vi "AutoHelper_Timeout.vi"(6 "Pass_Through_Time":dbl=-1.0 format="%33.4f", 9 "Timeout Sec":dbl, 11 "New Step":bool) -> (1 "Remaining":dbl, 3 "Timeout":bool)   [LabVIEW 2019, in "Trajectory_Library.lvlib"]
doc: "Implements a simplified state machine similar to a mechanical / electrical drum sequencer. When the Drum Sequencer is \"Ready\" and the \"Initiate\" input becomes TRUE,, the drum sequences through its set of steps from 1 to N. After each Step is executed it is followed by a wait. During the wait the Step output indicates \"Do Nothing\". The number of Steps is determined by the number of elements in the \"Step Times\" input array. Once all the steps have been executed, the Drum Sequencer cycles bac to wait for another initiate. \n\nThere is a Cancel input that interrupts the sequence, executes the Cancel Step, performs the cancel wait, and then returns to wait for an Initiate action. \n\nIf any of the Step Times, or Cancel times are negative, or there more than 32 steps, or less than 1 step an error is signaled. The drum sequencer selects the error state and stays there.\n\nInputs:\n\nOutputs:"
uses:
  Trajectory_Library.lvlib
  Util_GetTime_U32.vi
  Util_GetTime_U64.vi
  <vilib>/Utility/semaphor.llb/Obtain Semaphore Reference.vi
  Timer_Reset.vi
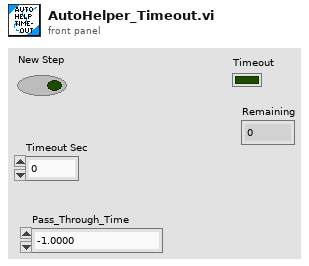
[diagram p1: front panel]
types:
  T1 = typedef "Trajectory_Library.lvlib/TIMER.ctl" = cluster{"StartTime":dbl, "Accumulated TIme":dbl, "Running":bool, "semaphore":T2}
  T2 = typedef "Semaphore RefNum" = refnum<k1>
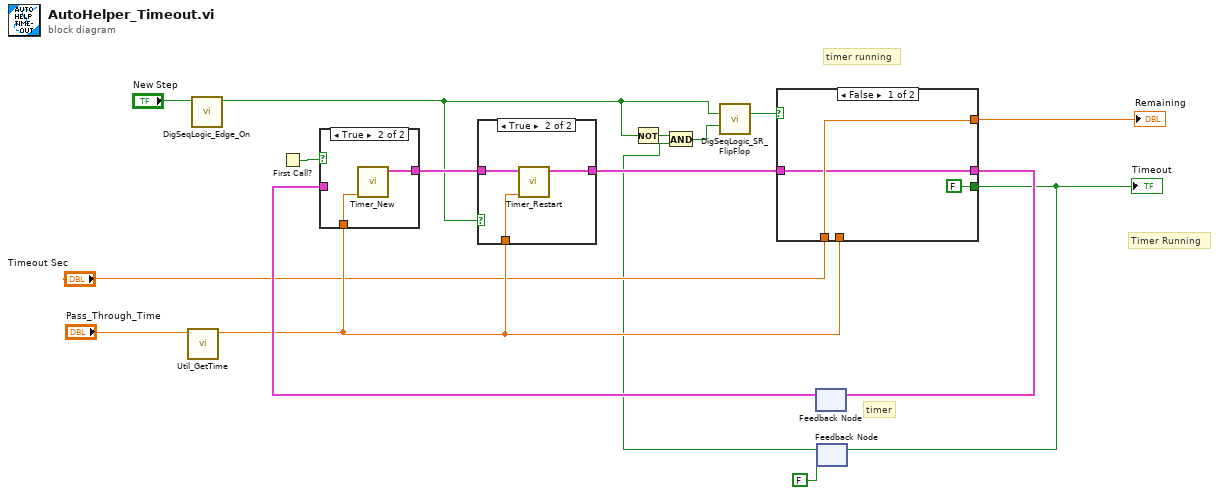
[diagram p0: block diagram]
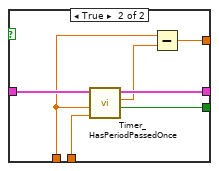
[diagram p2: hidden frame]
diagram:
  # "timer running"
  # "Timer Running"
  # "timer"
  n1 = call "Util_GetTime.vi"("Pass_Through_Time"="Pass_Through_Time") -> ("FPGA_Time_Seconds"=w11:dbl)  [unwired: 8 in, 2 out]
  n2 = call "DigSeqLogic_Edge_On.vi"("Input"="New Step") -> ("On Edge"=w5:bool)  [unwired: 10 in]
  n3 = First Call?() -> (First Call?: T/F=w15:bool)
  n4 = Not(x=w5) -> (.not. x?=w4:bool)
  n5 = feedback #1() -> (w14:T1)  [unwired: 1 in]
  n6 = case shown="True" w15 {
    tunnel: [w18 w20] -> w13
    tunnel: w11 -> [_ w19]
    tunnel: w14 -> [w18 _]
    frame False {
    }
    frame True {
      n7 = call "Timer_New.vi"("Pass_Through_Time"=w19) -> ("TIMER"=w20:T1)  [unwired: 10 in]
    }
  }
  n8 = case shown="True" w5 {
    tunnel: [w21 w24] -> w12
    tunnel: w13 -> [w21 w23]
    tunnel: w11 -> [_ w22]
    frame False {
    }
    frame True {
      n9 = call "Timer_Restart.vi"("Pass_Through_Time"=w22, "in Timer"=w23) -> ("out Timer"=w24:T1)  [unwired: 9 in]
    }
  }
  n10 = feedback #2(FALSE ("Expired")) -> (w2:bool)
  n11 = And(x=w4, y=w2) -> (x .and. y?=w3:bool)
  n12 = call "DigSeqLogic_SR_FlipFlop.vi"("Set"=w5, "Reset"=w3) -> ("Output"=w7:bool)  [unwired: 12 in, 1 out]
  n13 = case shown="False" w7 {
    tunnel: w12 -> [w26 w34]
    tunnel: w11 -> [_ w33]
    tunnel: [w26 w32] -> w10
    tunnel: "Timeout Sec" -> [w27 w31]
    tunnel: [w27 w29] -> w8
    tunnel: [FALSE ("Expired") w28] -> w6
    frame False {
    }
    frame True {
      n14 = call "Timer_HasPeriodPassedOnce.vi"("Pass_Through_Time"=w33, "Period"=w31, "in Timer"=w34) -> ("Expired"=w28:bool, "CurrentTImer"=w30:dbl, "out Timer"=w32:T1)  [unwired: 6 in]
      n15 = Subtract(x=w31, y=w30) -> (x-y=w29:dbl)
    }
  }
  "Timeout" <- w6
  "Remaining" <- w8
  n16 = feedback-in #1(w10) -> ()
  n17 = feedback-in #2(w6) -> ()
